vi "To Variant.vi"(0 "KObject in":refnum<class "KObject.lvclass">, 11 "error in (no error)":errorcluster) -> (4 "KObject out":refnum<class "KObject.lvclass">, 8 "Array":variant[](array[variant]), 15 "error out":errorcluster)   [LabVIEW 2020, in "KObject.lvclass"]
uses:
  KObject.lvclass
  KObject.lvclass/KObject.ctl
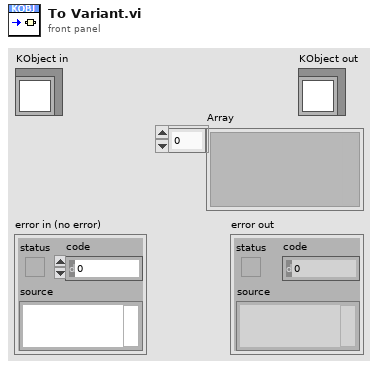
[diagram p1: front panel]
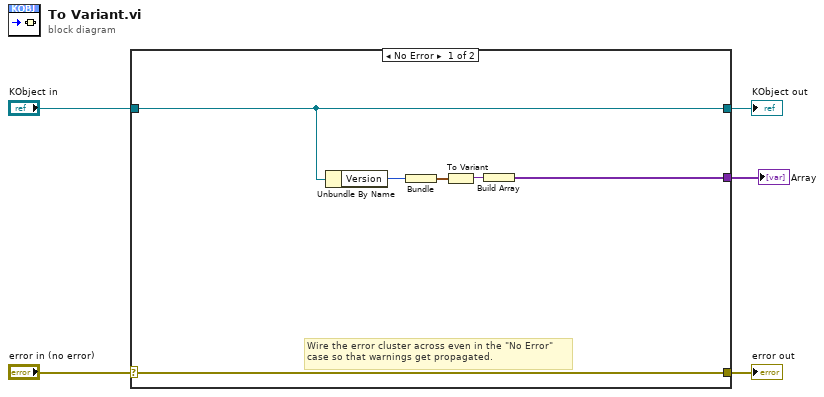
[diagram p0: block diagram]
diagram:
  n1 = case shown="No Error" "error in (no error)" {
    selector: "error in (no error)" -> [w11 w13]
    tunnel: [w11 w13] -> w4
    tunnel: [w8 w12] -> w2
    tunnel: "KObject in" -> [w8 w12]
    tunnel: [w9 _] -> w1
    frame No Error {
      # "Wire the error cluster across even in the \"No Error\"\ncase so that warnings get propagated."
      n2 = Unbundle By Name(w8) -> ("Version"=w7:i32)
      n3 = Bundle("Version"=w7) -> (w6:cluster{"Version":i32})  [unwired: 1 in]
      n4 = To Variant(anything=w6) -> (Variant=w10:variant)
      n5 = Build Array(w10) -> (w9:variant[])
    }
    frame Error {
    }
  }
  "error out" <- w4
  "KObject out" <- w2
  "Array" <- w1
